vi "J1939 Claim With Address.vi"(8 "error in (no error)":errorcluster, 9 "SAE J1939:Node Address":u8, 10 "SAE J1939:Node Name":u64, 11 "XNET Session":refnum<k21>) -> (0 "error out":errorcluster, 2 "Assigned J1939 Address":u8, 3 "XNET Session Out":refnum<k21>)   [LabVIEW 2013, in "J1939 runtime.lvclass"]
uses:
  J1939 runtime.lvclass
  <resource>/objmgr/xnet.rc
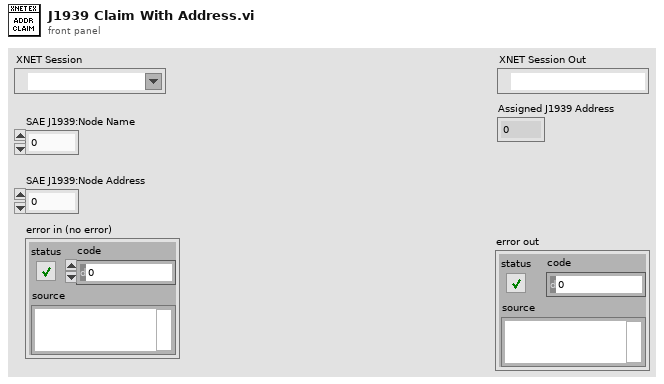
[diagram p1: front panel]
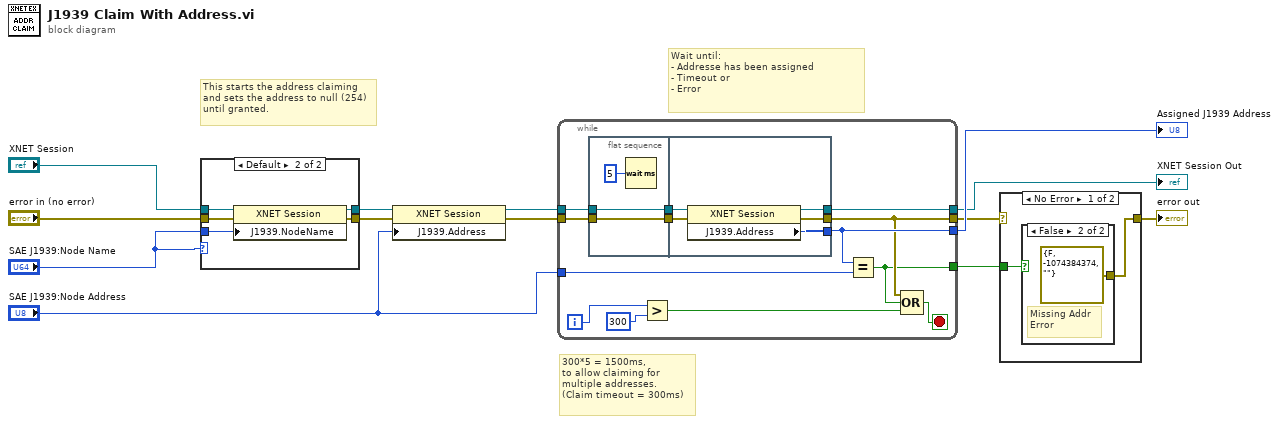
[diagram p0: block diagram]
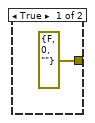
[diagram p3: hidden frame]
diagram:
  # "This starts the address claiming\nand sets the address to null (254)\nuntil granted."
  # "300*5 = 1500ms,\nto allow claiming for \nmultiple addresses.\n(Claim timeout = 300ms)"
  # "Wait until:\n- Addresse has been assigned\n- Timeout or\n- Error"
  n1 = case shown="Default" "SAE J1939:Node Name" {
    tunnel: "XNET Session" -> [w15 w20]
    tunnel: "SAE J1939:Node Name" -> [_ w19]
    tunnel: "error in (no error)" -> [w14 w18]
    tunnel: [w15 w17] -> w3
    tunnel: [w14 w16] -> w2
    frame 0 {
    }
    frame Default {
      n2 = property class="XNET Session"(reference=w20, error in=w18, "J1939.NodeName"=w19) -> (reference out=w17:refnum<k21>, error out=w16:errorcluster)
    }
  }
  n3 = property class="XNET Session"(reference=w3, error in=w2, "J1939.Address"="SAE J1939:Node Address") -> (reference out=w11:refnum<k21>, error out=w12:errorcluster)
  n4 = while {
    tunnel: [w31] -> w13
    tunnel: w12 -> [w33]
    tunnel: [w25] -> w8
    tunnel: w11 -> [w30]
    tunnel: [w28] -> w10
    tunnel: "SAE J1939:Node Address" -> [w22]
    tunnel: [w21] -> w9
    i -> [w27]
    stop <- w24 stop-if-true
    n5 = flat-sequence {
      tunnel: w33 -> [w36]
      tunnel: [w36] -> w32
      tunnel: w30 -> [w34]
      tunnel: [w34] -> w29
      tunnel: [w41] -> w31
      tunnel: w32 -> [w40]
      tunnel: [w39] -> w25
      tunnel: w29 -> [w38]
      tunnel: [w37] -> w28
      frame #0 {
        n6 = Wait (ms)(milliseconds to wait=u32 5) -> ()  [unwired: 1 out]
      }
      frame #1 {
        n7 = property class="XNET Session"(reference=w38, error in=w40) -> (reference out=w37:refnum<k21>, error out=w39:errorcluster, "J1939.Address"=w41:u8)
      }
    }
    n8 = Greater?(x=w27, y=300) -> (0:w23:bool)
    n9 = Equal?(x=w31, y=w22) -> (x = y?=w21:bool)
    n10 = Compound Arithmetic op=OR(w25, w21, w23) -> (w24:bool)
  }
  "Assigned J1939 Address" <- w13
  "XNET Session Out" <- w10
  n11 = case shown="No Error" w8 {
    selector: w8 -> [_ w46]
    tunnel: w9 -> [w43 _]
    tunnel: [w42 w46] -> w7
    frame No Error {
      n12 = case shown="False" w43 {
        tunnel: [errorcluster {"status"=FALSE, "code"=0, "source"=""} ("error out") errorcluster {"status"=FALSE, "code"=-1074384374, "source"=""} ("error out")] -> w42
        frame True {
        }
        frame False {
          # "Missing Addr\nError"
        }
      }
    }
    frame Error {
    }
  }
  "error out" <- w7
